vi "Send File.vi"(8 "error in (no error)":errorcluster, 10 "Send File":bool, 11 "Logger in.lvclass":refnum<class "Logger.lvclass">) -> (0 "error out":errorcluster, 1 "File Sent":bool, 2 "Files Sent":i32, 3 "Logger out.lvclass":refnum<class "Logger.lvclass">)   [LabVIEW 2017, in "Logger.lvclass"]
uses:
  Logger.lvclass
  Logger.lvclass/Logger.ctl
  <vilib>/Skyline/Message/NI Skyline Message (Sync).lvclass
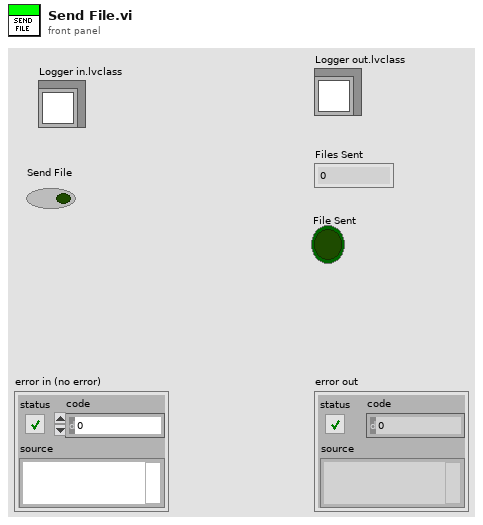
[diagram p1: front panel]
types:
  T1 = cluster{"Tag Units":string, "Tag Path":string, "Waveform":waveform(dbl), "Log":bool, "Tag Reference":refnum<class "NI Skyline Tag.lvclass">}[]
  T2 = cluster{"Tag Units":string, "Tag Path":string, "Waveform":waveform(dbl), "Log":bool, "Tag Reference":refnum<class "NI Skyline Tag.lvclass">}
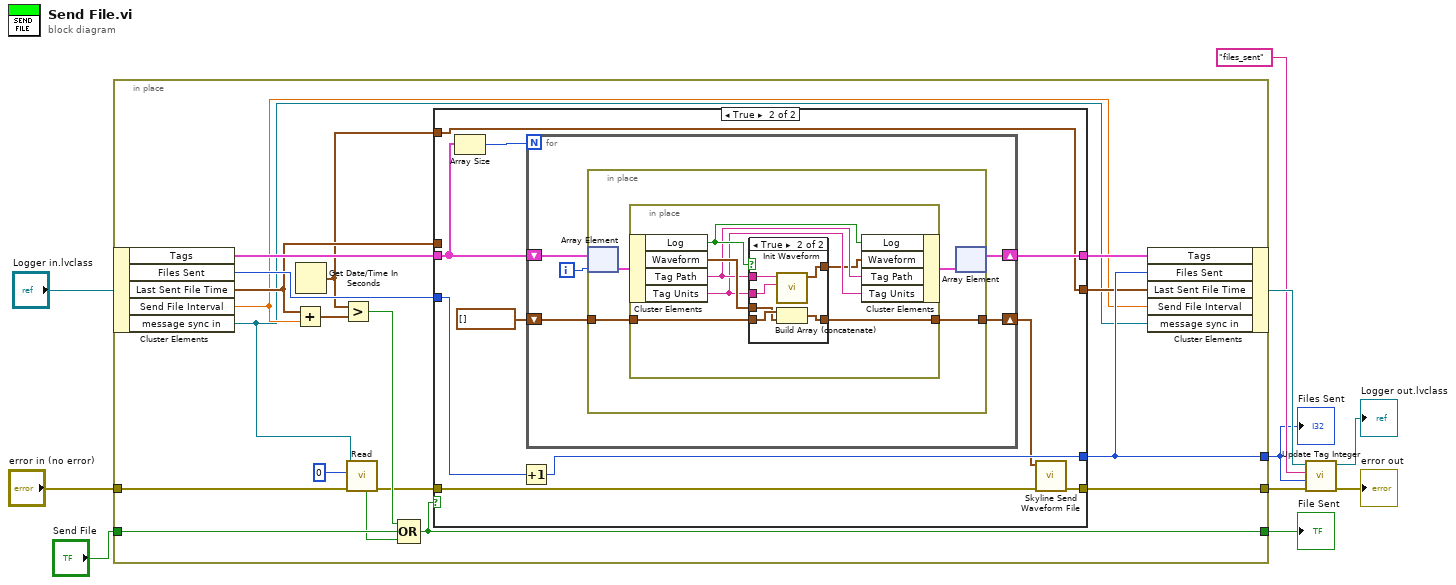
[diagram p0: block diagram]
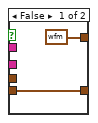
[diagram p3: hidden frame]
diagram:
  n1 = in-place {
    in-place-border: [w25] -> w1
    in-place-border: "Send File" -> [w23]
    in-place-border: [w19] -> w3
    in-place-border: [w18] -> w8
    in-place-border: "error in (no error)" -> [w16]
    n2 = in-place-cluster #1("Logger in.lvclass") -> ("Tags"=w27:T1, "Files Sent"=w26:i32, "Last Sent File Time"=w21:timestamp, "Send File Interval"=w20:dbl, "message sync in"=w11:refnum<class "NI Skyline Message (Sync).lvclass">)
    n3 = Add(x=w21, y=w20) -> (x+y=w12:timestamp)
    n4 = Get Date/Time In Seconds() -> (seconds since 1Jan1904=w13:timestamp)
    n5 = Greater?(x=w13, y=w12) -> (0:w24:bool)
    n6 = call <vilib>:"Read.vi"("error in (no error)"=w16, "timeout milliseconds (100)"=0 ("timeout milliseconds"), "message sync in"=w11) -> ("error out"=w17:errorcluster, "dequeue status"=w14:bool)  [unwired: 4 in, 3 out]
    n7 = Compound Arithmetic op=OR(w24, w23, w14) -> (w18:bool)
    n8 = case shown="True" w18 {
      tunnel: [w31 w42] -> w28
      tunnel: w27 -> [w31 w40]
      tunnel: w26 -> [w32 w39]
      tunnel: [w32 w38] -> w25
      tunnel: [w30 w36] -> w22
      tunnel: w21 -> [w30 _]
      tunnel: w13 -> [_ w36]
      tunnel: w17 -> [w29 w35]
      tunnel: [w29 w34] -> w19
      frame False {
      }
      frame True {
        n9 = Array Size(array=w40) -> (size(s)=w41:i32)
        n10 = Increment(x=w39) -> (x+1=w38:i32)
        n11 = for {
          N: w41 -> [_]
          shift-right: [w45] -> w42
          shift-left: w40 -> [w47]
          shift-right: [w43] -> w37
          shift-left: waveform(dbl)[] [] -> [w44]
          i -> [w46]
          n12 = in-place {
            in-place-border: w44 -> [w49]
            in-place-border: [w48] -> w43
            n13 = in-place-array #2(w47, w46) -> (w50:T2)
            n14 = in-place {
              in-place-border: w49 -> [w58]
              in-place-border: [w56] -> w48
              n15 = in-place-cluster #3(w50) -> ("Log"=w55:bool, "Waveform"=w57:waveform(dbl), "Tag Path"=w54:string, "Tag Units"=w53:string)
              n16 = case shown="True" w55 {
                tunnel: w58 -> [w60 w66]
                tunnel: w57 -> [_ w65]
                tunnel: [w60 w64] -> w56
                tunnel: w54 -> [_ w63]
                tunnel: w53 -> [_ w62]
                tunnel: [waveform(dbl) {"t0"=timestamp(0 s since 1904-01-01), "dt"=1.0, "Y"=[]} ("waveform") w61] -> w52
                frame False {
                }
                frame True {
                  n17 = call "Init Waveform.vi"("Units"=w62, "System Tag"=w63) -> ("waveform"=w61:waveform(dbl))  [unwired: 8 in, 1 out]
                  n18 = Build Array (concatenate)(w66, w65) -> (w64:waveform(dbl)[])
                }
              }
              n19 = in-place-cluster #3("Log"=w55, "Waveform"=w52, "Tag Path"=w54, "Tag Units"=w53) -> (w51:T2)
            }
            n20 = in-place-array #2(w51) -> (w45:T1)  [unwired: 1 out]
          }
        }
        n21 = call "Skyline Send Waveform File.vi"("error in"=w35, "data in"=w37) -> ("error out"=w34:errorcluster)  [unwired: 8 in, 1 out]
      }
    }
    n22 = in-place-cluster #1("Tags"=w28, "Files Sent"=w25, "Last Sent File Time"=w22, "Send File Interval"=w20, "message sync in"=w11) -> (w5:refnum<class "Logger.lvclass">)
  }
  "Files Sent" <- w1
  "File Sent" <- w8
  n23 = call "Update Tag Integer.vi"("error in (no error)"=w3, "Value"=w1, "Tag Path"="files_sent", "Logger in.lvclass"=w5) -> ("error out"=→"error out":errorcluster, "Logger out.lvclass"=→"Logger out.lvclass":refnum<class "Logger.lvclass">)  [unwired: 6 in]
